vi "Hormiga_Init.vi"(3 "error in (no error)":errorcluster, 4 "Velocidad de Conexion":enum16{"115200", "9600"}(ring), 5 "VISA Refnum in":refnum<visa-resource-name>) -> (0 "error out":errorcluster, 2 "VISA Refnum out":refnum<visa-resource-name>)   [LabVIEW 2016]
uses:
  <vilib>/Instr/_visa.llb/VISA Find Search Mode.ctl
  <vilib>/Instr/_visa.llb/VISA Configure Serial Port (Instr).vi
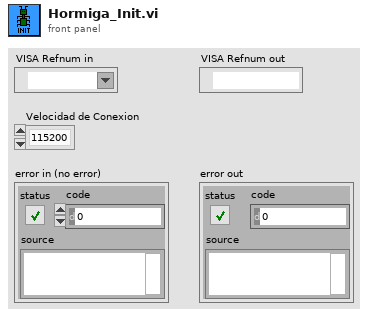
[diagram p1: front panel]
types:
  T1 = typedef "VISA Find Search Mode.ctl" = u32
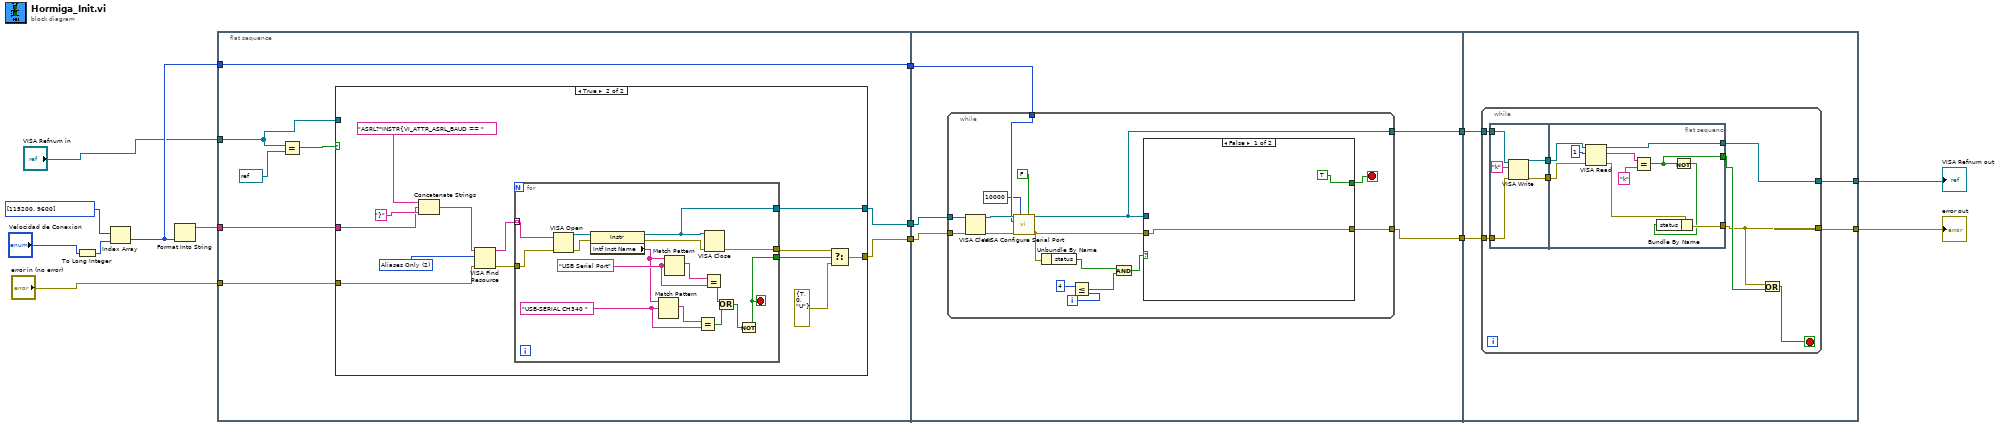
[diagram p0: block diagram]
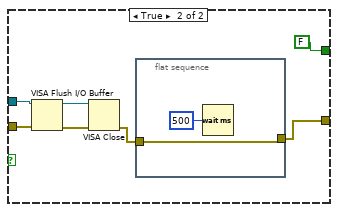
[diagram p3: hidden frame]
diagram:
  n1 = To Long Integer(number="Velocidad de Conexion") -> (32bit integer=w5:i32)
  n2 = Index Array(array=u32[] [115200, 9600], index=w5) -> (element=w2:u32)
  n3 = Format Into String(w2) -> (resulting string=w3:string)  [unwired: 3 in, 1 out]
  n4 = flat-sequence {
    tunnel: "VISA Refnum in" -> [w20]
    tunnel: "error in (no error)" -> [w19]
    tunnel: w3 -> [w18]
    tunnel: w2 -> [w15]
    tunnel: [w17] -> w14
    tunnel: [w16] -> w13
    tunnel: [w15] -> w12
    tunnel: w14 -> [w56]
    tunnel: w13 -> [w57]
    tunnel: w12 -> [w58]
    tunnel: [w55] -> w11
    tunnel: [w54] -> w10
    tunnel: w11 -> [w87]
    tunnel: w10 -> [w88]
    tunnel: [w89] -> w8
    tunnel: [w86] -> w9
    frame #0 {
      n5 = Equal?(x=w20, y=refnum<visa-resource-name> refnum ("VISA resource name 2")) -> (x = y?=w21:bool)
      n6 = case shown="True" w21 {
        tunnel: [w24 w28] -> w16
        tunnel: w20 -> [w23 _]
        tunnel: w19 -> [w24 w27]
        tunnel: [w23 w26] -> w17
        tunnel: w18 -> [_ w25]
        frame False {
        }
        frame True {
          w37 = T1 2 items=["Canonical Names Only"=0, "Aliases Only"=2, "Include Matching Aliases"=3, "Include All Aliases"=4] ("Search Mode")
          n7 = Concatenate Strings("ASRL?*INSTR{VI_ATTR_ASRL_BAUD == " ("string"), w25, "}" ("string")) -> (w32:string)
          n8 = VISA Find Resource(8:w27, 10:w37, 11:w32) -> (0:w35:errorcluster, 3:w36:string[])  [unwired: 1 out]
          n9 = for {
            tunnel: w36 -> [w52] mode=indexing
            tunnel: w35 -> [w53]
            tunnel: [w47] -> w26
            tunnel: [w45] -> w31
            tunnel: [w38] -> w29
            stop <- w38 stop-if-true
            w43 = "USB-SERIAL CH340 " ("regular expression")
            w48 = "USB Serial Port" ("regular expression")
            n10 = VISA Open(error in (no error)=w53, VISA resource name=w52) -> (VISA resource name=w51:refnum<visa-resource-name>, error out=w50:errorcluster)  [unwired: 3 in]
            n11 = property class="Instr"(reference=w51, error in=w50) -> (reference out=w47:refnum<visa-resource-name>, error out=w46:errorcluster, "Intf Inst Name"=w42:string)
            n12 = Match Pattern(string=w42, regular expression=w43) -> (match substring=w44:string)  [unwired: 1 in, 3 out]
            n13 = Match Pattern(string=w42, regular expression=w48) -> (match substring=w49:string)  [unwired: 1 in, 3 out]
            n14 = Equal?(x=w44, y=w43) -> (x = y?=w41:bool)
            n15 = Equal?(x=w49, y=w48) -> (x = y?=w40:bool)
            n16 = VISA Close(VISA resource name=w47, error in (no error)=w46) -> (error out=w45:errorcluster)
            n17 = Or(x=w40, y=w41) -> (x .or. y?=w39:bool)
            n18 = Not(x=w39) -> (.not. x?=w38:bool)
          }
          n19 = Select(t=w31, s=w29, f=errorcluster {"status"=TRUE, "code"=0, "source"="U"} ("error out")) -> (s? t:f=w28:errorcluster)
        }
      }
    }
    frame #1 {
      n20 = while {
        tunnel: w58 -> [w72]
        tunnel: w56 -> [w69]
        tunnel: w57 -> [w68]
        tunnel: [w61] -> w54
        tunnel: [w60] -> w55
        i -> [w67]
        stop <- w62 stop-if-true
        n21 = VISA Clear(VISA resource name=w69, error in (no error)=w68) -> (VISA resource name out=w74:refnum<visa-resource-name>, error out=w73:errorcluster)
        n22 = call-poly "VISA Configure Serial Port"("VISA resource name"=w74, "timeout (10sec)"=u32 10000, "Enable Termination\nChar (T)"=FALSE ("Enable Termination\nChar (T)"), "baud rate (9600)"=w72, "error in (no error)"=w73) -> ("VISA resource name out"=w60:refnum<visa-resource-name>, "error out"=w63:errorcluster)  [unwired: 9 in]
        n23 = Unbundle By Name(w63) -> ("status"=w59:bool)
        n24 = Less Or Equal?(x=4, y=w67) -> (x <= y?=w65:bool)
        n25 = And(x=w59, y=w65) -> (x .and. y?=w64:bool)
        n26 = case shown="False" w64 {
          tunnel: w63 -> [w75 w83]
          tunnel: w60 -> [_ w82]
          tunnel: [TRUE FALSE] -> w62
          tunnel: [w75 w77] -> w61
          frame False {
          }
          frame True {
            n27 = VISA Flush I/O Buffer(VISA resource name=w82, error in (no error)=w83) -> (VISA resource name out=w80:refnum<visa-resource-name>, error out=w81:errorcluster)  [unwired: 1 in]
            n28 = VISA Close(VISA resource name=w80, error in (no error)=w81) -> (error out=w78:errorcluster)
            n29 = flat-sequence {
              tunnel: [w84] -> w77
              tunnel: w78 -> [w84]
              frame #0 {
                n30 = Wait (ms)(milliseconds to wait=u32 500) -> ()  [unwired: 1 out]
              }
            }
          }
        }
      }
    }
    frame #2 {
      n31 = while {
        tunnel: [w90] -> w89
        tunnel: w88 -> [w97]
        tunnel: w87 -> [w96]
        tunnel: [w93] -> w86
        stop <- w92 stop-if-true
        n32 = flat-sequence {
          tunnel: w97 -> [w99]
          tunnel: w96 -> [w98]
          tunnel: [w101] -> w95
          tunnel: [w100] -> w94
          tunnel: w95 -> [w106]
          tunnel: w94 -> [w107]
          tunnel: [w108] -> w90
          tunnel: [w105] -> w93
          tunnel: [w103] -> _
          tunnel: [w103] -> w91
          frame #0 {
            n33 = VISA Write(VISA resource name=w98, write buffer="k", error in (no error)=w99) -> (VISA resource name out=w101:refnum<visa-resource-name>, error out=w100:errorcluster)  [unwired: 1 out]
          }
          frame #1 {
            n34 = VISA Read(VISA resource name=w106, byte count=u32 1, error in (no error)=w107) -> (VISA resource name out=w105:refnum<visa-resource-name>, read buffer=w112:string, error out=w109:errorcluster)  [unwired: 1 out]
            n35 = Equal?(x=w112, y="k") -> (x = y?=w103:bool)
            n36 = Not(x=w103) -> (.not. x?=w104:bool)
            n37 = Bundle By Name(cluster=w109, "status"=w104) -> (w108:errorcluster)
          }
        }
        n38 = Or(x=w90, y=w91) -> (x .or. y?=w92:bool)
      }
    }
  }
  "VISA Refnum out" <- w9
  "error out" <- w8
